vi "niRFSGPlayback Generate Waveform.vi"(6 "instrument handle":refnum<k15>, 7 "Port":string, 8 "error in (no error)":errorcluster, 9 "LO configure setting":T1={"Carrier Frequency (Hz)"=5180000000.0, "Power Level(dBm)"=-10.0, "External Attenuation (dB)"=0.0} {"Carrier Frequency (Hz)" format="%#_6p"}, 10 "TX port":string="port1", 11 "TSM Context":T2) -> (0 "error out":errorcluster {"code" format="%.0x"}, 1 "instrument handle out":refnum<k15>)   [LabVIEW 2014]
doc: "This example demonstrates generation of 802.11 single-channel waveform using an NI vector signal generator. The example reads the waveform from a TDMS file."
uses:
  <vilib>/NI_TestStand_SemiconductorModule/NI_TestStand_Semiconductor_Module.lvlibp/PinMap/General/SemiconductorModuleContext.ctl
  <vilib>/NI_TestStand_SemiconductorModule/NI_TestStand_Semiconductor_Module.lvlibp/PinMap/RF/RFSG/PinToNIRFSGSession.vi
  <instrlib>/niRFPM/niRFPM.llb/NI-RFPM Set TX Path By Parameters.vi
  <instrlib>/niRFPM/niRFPM.llb/NI-RFPM Fetch Source Offset By Parameters.vi
  <vilib>/NI_TestStand_SemiconductorModule/NI_TestStand_Semiconductor_Module.lvlibp
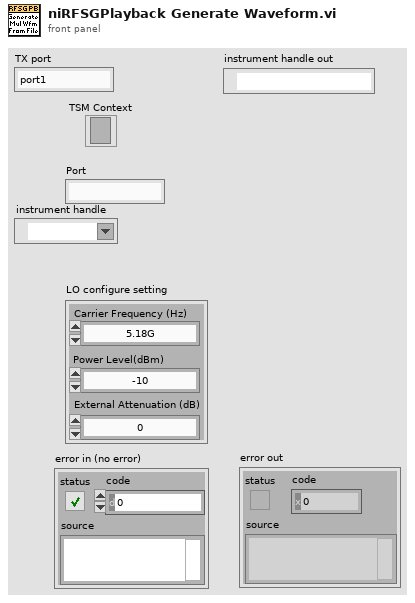
[diagram p1: front panel]
types:
  T1 = cluster{"Carrier Frequency (Hz)":dbl, "Power Level(dBm)":dbl, "External Attenuation (dB)":dbl}
  T2 = typedef "NI_TestStand_Semiconductor_Module.lvlibp/SemiconductorModuleContext.ctl" = refnum<k7>
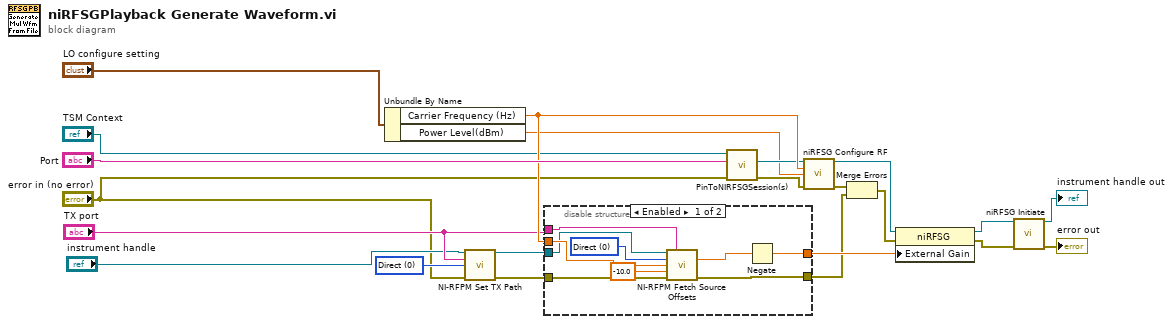
[diagram p0: block diagram]
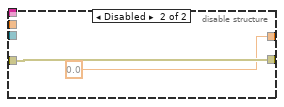
[diagram p2: hidden frame]
diagram:
  w19 = 0 items=["Direct", "Gain", "Loop"] ("TX Path")
  n1 = Unbundle By Name("LO configure setting") -> ("Carrier Frequency (Hz)"=w17:dbl, "Power Level(dBm)"=w3:dbl)
  n2 = call-poly <instrlib>:"NI-RFPM Set TX Path.vi"("instrument handle"="instrument handle", "TX port"="TX port", "TX Path"=w19, "error in (no error)"="error in (no error)") -> ("instrument handle out"=w16:refnum<k15>, "error out"=w8:errorcluster)  [unwired: 10 in]
  n3 = disable-structure shown="Enabled" {
    disable-tunnel: w8 -> [w31 w33]
    disable-tunnel: [w24 0.0] -> w18
    disable-tunnel: [w30 w33] -> w4
    disable-tunnel: w17 -> [w29 _]
    disable-tunnel: w16 -> [w27 _]
    disable-tunnel: "TX port" -> [w26 _]
    frame Enabled {
      w28 = u32 0 items=["Unspecified"=3, "Loop"=2, "Gain"=1, "Direct"=0] ("Source Path")
      n4 = call-poly <instrlib>:"NI-RFPM Fetch Source Offsets.vi"("instrument handle"=w27, "Port"=w26, "Source Path"=w28, "frequency"=w29, "power"=-10.0, "error in"=w31) -> ("SourceOffset"=w25:dbl, "error out"=w30:errorcluster)  [unwired: 6 in, 2 out]
      n5 = Negate(x=w25) -> (-x=w24:dbl)
    }
    frame Disabled {
    }
  }
  n6 = call-poly <vilib>:"PinToNIRFSGSession(s).vi"("error in (no error)"="error in (no error)", "Pin"="Port", "Semiconductor Module Context"="TSM Context") -> ("error out"=w10:errorcluster, "Instrument Session"=w11:refnum<k15>)  [unwired: 5 in, 2 out]
  n7 = call <instrlib>:"niRFSG Configure RF.vi"("instrument handle"=w11, "frequency (Hz)"=w17, "power level (dBm)"=w3, "error in"=w10) -> ("instrument handle out"=w21:refnum<k15>, "error out"=w5:errorcluster)  [unwired: 10 in]
  n8 = Merge Errors(w5, w4) -> (w6:errorcluster)
  n9 = property class="niRFSG"(reference=w21, error in=w6, "External Gain"=w18) -> (reference out=w1:refnum<k15>, error out=w2:errorcluster)
  n10 = call <instrlib>:"niRFSG Initiate.vi"("instrument handle"=w1, "error in"=w2) -> ("instrument handle out"=→"instrument handle out":refnum<k15>, "error out"=→"error out":errorcluster)  [unwired: 12 out]
